vi "Read Test Suite Results.vi"(8 "error in (no error)":errorcluster, 11 "Report In":refnum<class "Test Report.lvclass">) -> (0 "error out":errorcluster, 2 "Test Suite Results":T1[](array[typedef]), 3 "Report Out":refnum<class "Test Report.lvclass">)   [LabVIEW 2020, in "Test Report.lvclass"]
uses:
  Test Report.lvclass
  Result Types/Suite Results/Test Suite Result.ctl
  Result Types/Assertion Result/Public/TypeDefs/Status.ctl
  Result Types/Case Result/Test Case Result.ctl
  Result Types/Method Result/Method Result.ctl
  Result Types/Assertion Result/Assertion Result.ctl
  Result Types/Assertion Result/Public/TypeDefs/Assertion Type.ctl
  Test Report.lvclass/Test Report.ctl
  Result Types/Assertion Result/Assertion Result.lvlib
  Result Types/Method Result/Method Result.lvlib
  Result Types/Case Result/Test Case Result.lvlib
  Result Types/Suite Results/Test Suite Result.lvlib
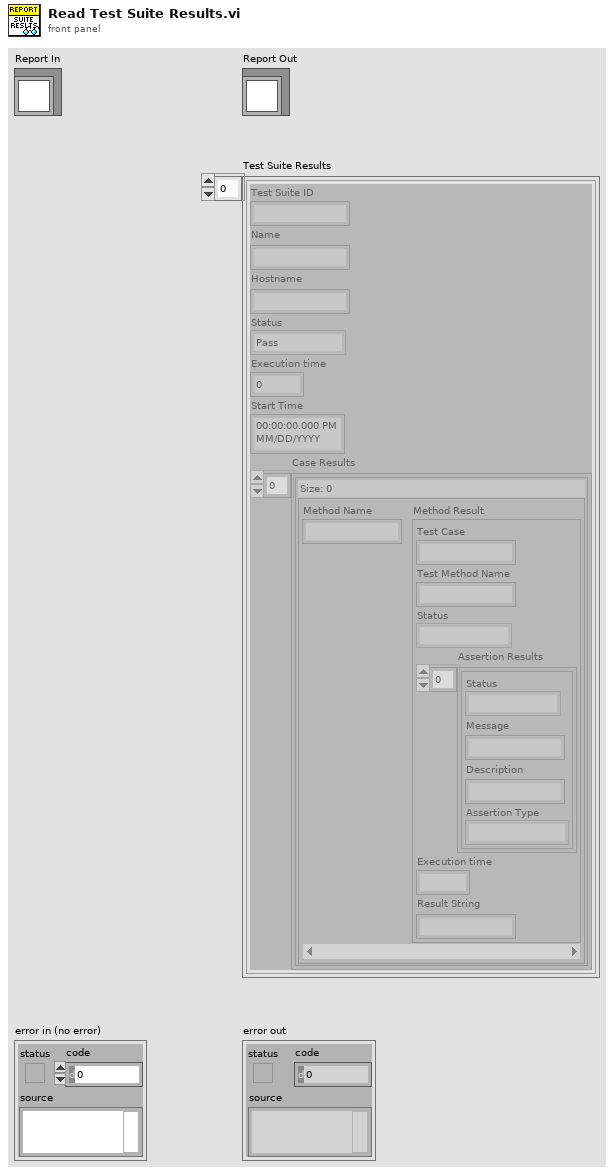
[diagram p1: front panel]
types:
  T1 = typedef "Test Suite Result.lvlib/Test Suite Result.ctl" = cluster{"Test Suite ID":string, "Name":string, "Hostname":string, "Status":T2, "Execution time":dbl, "Start Time":timestamp, "Case Results":T3[]}
  T2 = typedef "Assertion Result.lvlib/Status.ctl" = enum16{"Pass", "Fail", "Error", "Skipped", "Setup Error", "Broken", "Teardown Error"}
  T3 = typedef "Test Case Result.lvlib/Test Case Result.ctl" = map{string, T4}
  T4 = typedef "Method Result.lvlib/Method Result.ctl" = cluster{"Test Case":string, "Test Method Name":string, "Status":T2, "Assertion Results":T5[], "Execution time":dbl, "Result String":string}
  T5 = typedef "Assertion Result.lvlib/Assertion Result.ctl" = cluster{"Status":T2, "Message":string, "Description":string, "Assertion Type":T6}
  T6 = typedef "Assertion Result.lvlib/Assertion Type.ctl" = enum16{"None", "Pass", "Fail", "Skip", "Pass if Equal", "Fail if Equal", "Pass if Error", "Fail if Error", "Pass if", "Fail if"}
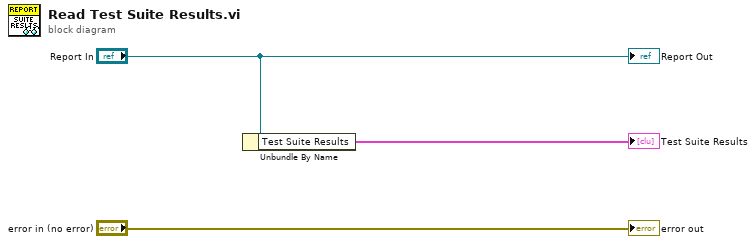
[diagram p0: block diagram]
diagram:
  n1 = Unbundle By Name("Report In") -> ("Test Suite Results"=→"Test Suite Results":T1[])
  "error out" <- "error in (no error)"
  "Report Out" <- "Report In"
